vi "Reflect Points.vi"(4 "Scaling Vector":cluster{dbl, dbl}, 5 "Arc Point Arrays":cluster{dbl[], dbl[], dbl[]}, 6 "Blend Point Arrays":cluster{dbl[], dbl[], dbl[]}, 7 "Blend Exit Point":cluster{dbl, dbl}, 8 "Extra Arc rad":dbl, 9 "Delta Points":cluster{dbl, dbl}[](array[cluster]), 10 "Tangent Angle (rad)":dbl, 11 "Angle":dbl) -> (3 "Point Arrays":cluster{dbl[], dbl[], dbl[]})   [LabVIEW 2020]
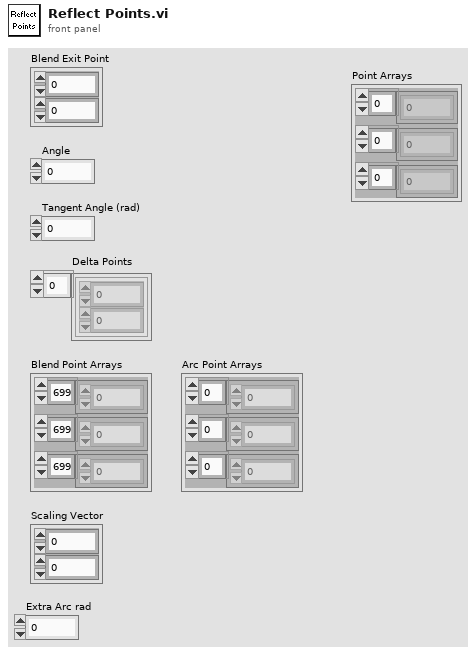
[diagram p1: front panel]
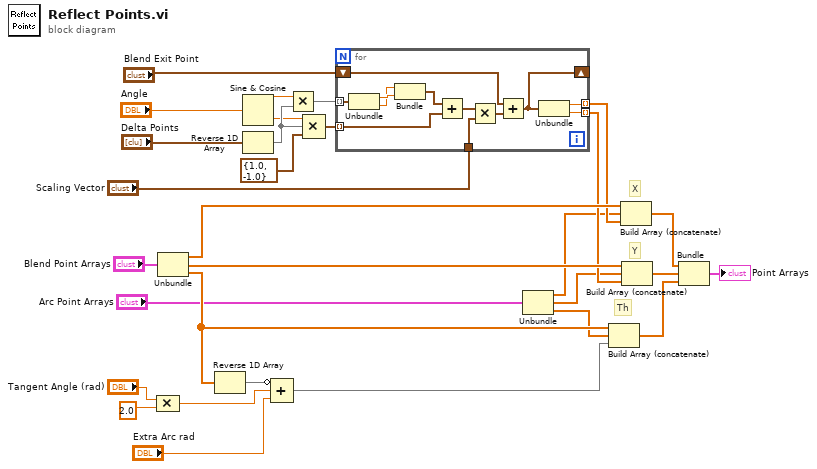
[diagram p0: block diagram]
diagram:
  # "Th"
  # "Y"
  # "X"
  n1 = Compound Arithmetic op=MULTIPLY("Tangent Angle (rad)", 2.0) -> (w2:dbl)
  n2 = Unbundle("Blend Point Arrays") -> (w10:dbl[], w13:dbl[], w15:dbl[])
  n3 = Reverse 1D Array(array=w15) -> (reversed array=w27:dbl[])
  n4 = Sine & Cosine(0:"Angle") -> (1:w17:dbl, 2:w16:dbl)
  n5 = Reverse 1D Array(array="Delta Points") -> (reversed array=w18:cluster{dbl, dbl}[])
  n6 = Compound Arithmetic op=ADD(invert w27, w2, "Extra Arc rad") -> (w7:dbl[])
  n7 = Multiply(x=w17, y=w18) -> (x*y=w19:cluster{dbl, dbl}[])
  n8 = Compound Arithmetic op=MULTIPLY(w16, w18, cluster{dbl, dbl} {1.0, -1.0}) -> (w20:cluster{dbl, dbl}[])
  n9 = for {
    tunnel: w19 -> [w40] mode=indexing
    tunnel: w20 -> [w38] mode=indexing
    shift-right: [w31] -> _
    shift-left: "Blend Exit Point" -> [w37]
    tunnel: [w36] -> w9 mode=indexing
    tunnel: [w35] -> w8 mode=indexing
    tunnel: "Scaling Vector" -> [w34]
    n10 = Unbundle(w40) -> (w42:dbl, w41:dbl)
    n11 = Bundle(w41, w42) -> (w39:cluster{dbl, dbl})  [unwired: 1 in]
    n12 = Add(x=w39, y=w38) -> (x+y=w33:cluster{dbl, dbl})
    n13 = Multiply(x=w33, y=w34) -> (x*y=w32:cluster{dbl, dbl})
    n14 = Add(x=w37, y=w32) -> (x+y=w31:cluster{dbl, dbl})
    n15 = Unbundle(w31) -> (w36:dbl, w35:dbl)
  }
  n16 = Unbundle("Arc Point Arrays") -> (w5:dbl[], w4:dbl[], w3:dbl[])
  n17 = Build Array (concatenate)(w15, w3, w7) -> (w14:dbl[])
  n18 = Build Array (concatenate)(w10, w5, w9) -> (w12:dbl[])
  n19 = Build Array (concatenate)(w13, w4, w8) -> (w11:dbl[])
  n20 = Bundle(w12, w11, w14) -> (→"Point Arrays":cluster{dbl[], dbl[], dbl[]})  [unwired: 1 in]
